vi "VirtualBench_IV Curve (PWS and DMM).vi"() -> ()   [LabVIEW 2015]
doc: "This example demonstrates a voltage sweep and a measurement of the current across the DUT to create an I-V curve."
uses:
  <vilib>/Utility/error.llb/DialogType.ctl
  <vilib>/VirtualBench/_DMM Configure Measurement4.vi
  <vilib>/VirtualBench/_PS Configure Voltage Output0.vi
  <vilib>/VirtualBench/VirtualBench.lvlib
panel:
  in  "Auto Range":i32(ring) items=["Low", "High"]
  in  "PWS Channel":tag="ps/+6V" caption="Channel"
  in  "Current Limit (A)":dbl=0.5 caption="Current Limit (no change)"
  in  "End Voltage (V)":dbl=5.0 caption="Frequency (no change)"
  in  "Start Voltage (V)":dbl caption="Frequency (no change)"
  in  "Number of Steps":i32=10
  in  "VirtualBench Device":tag="VB8012"
  out "Analog Data":cluster{dbl[], dbl[]}(graph)
  # "Power Supply Settings"
  # "DMM Settings"
  # "IV Curve"
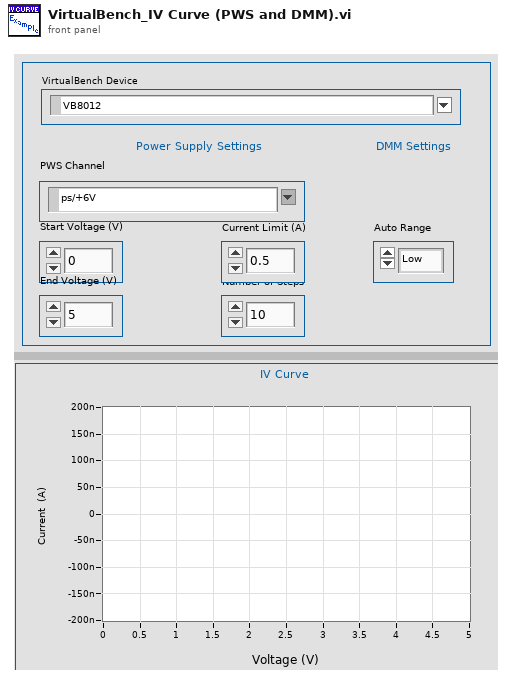
[diagram p1: front panel]
types:
  T1 = typedef "DialogType.ctl" = u16
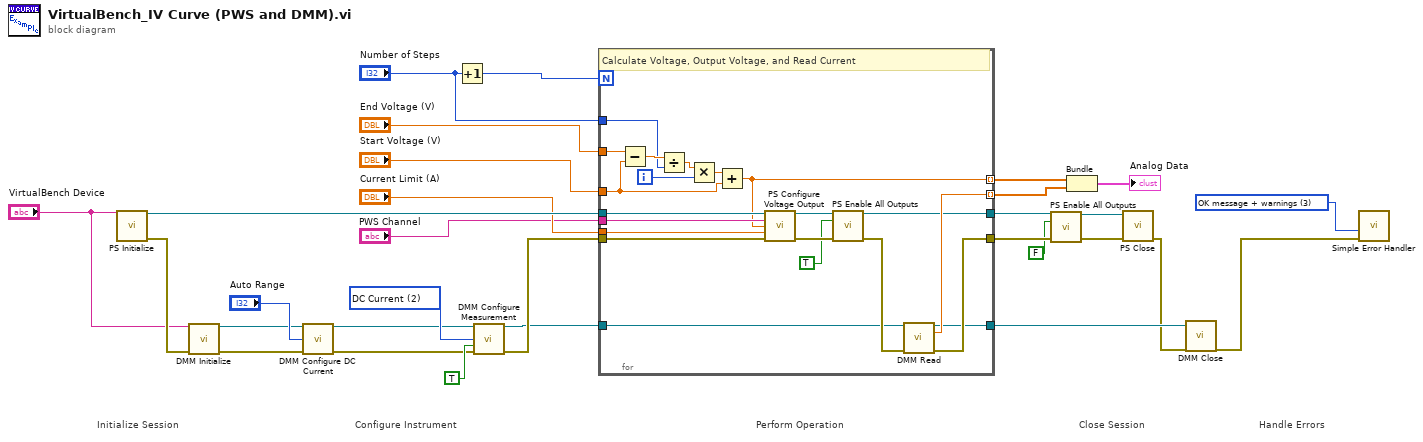
[diagram p0: block diagram]
diagram:
  w12 = 2 items=["DC Volts", "AC Volts", "DC Current", "AC Current", "Resistance", "Diode"] ("Function")
  w29 = T1 3 items=["no dialog", "OK message", "continue or stop message", "OK message + warnings", "continue/stop + warnings"] ("type of dialog (OK msg:1)")
  # "Handle Errors"
  # "Close Session"
  # "Configure Instrument"
  # "Perform Operation"
  # "Initialize Session"
  n1 = call <vilib>:"PS Initialize.vi"("Device Name"="VirtualBench Device") -> ("Instrument Handle Out"=w28:refnum<k21>, "Error Out"=w13:errorcluster)  [unwired: 13 in]
  n2 = call <vilib>:"DMM Initialize.vi"("Device Name"="VirtualBench Device", "Error In"=w13) -> ("Instrument Handle Out"=w1:refnum<k21>, "Error Out"=w2:errorcluster)  [unwired: 12 in]
  n3 = call <vilib>:"DMM Configure DC Current.vi"("Instrument Handle In"=w1, "Auto Range Terminal"="Auto Range", "Error In"=w2) -> ("Instrument Handle Out"=w4:refnum<k21>, "Error Out"=w3:errorcluster)  [unwired: 11 in]
  n4 = Increment(x="Number of Steps") -> (x+1=w30:i32)
  n5 = call-poly <vilib>:"DMM Configure Measurement.vi"("Instrument Handle In"=w4, "Function"=w12, "Auto Range"=TRUE, "Error In"=w3) -> ("Instrument Handle Out"=w7:refnum<k21>, "Error Out"=w14:errorcluster)  [unwired: 10 in]
  n6 = for {
    N: w30 -> [_]
    tunnel: "End Voltage (V)" -> [w48]
    tunnel: "Start Voltage (V)" -> [w47]
    tunnel: w28 -> [w45]
    tunnel: "Current Limit (A)" -> [w44]
    tunnel: "PWS Channel" -> [w40]
    tunnel: [w35] -> w19
    tunnel: [w37] -> w23 mode=indexing
    tunnel: w14 -> [w43]
    tunnel: [w33] -> w18
    tunnel: [w36] -> w22 mode=indexing
    tunnel: "Number of Steps" -> [w38]
    tunnel: [w32] -> w10
    tunnel: w7 -> [w31]
    i -> [w46]
    # "Calculate Voltage, Output Voltage, and Read Current"
    n7 = Subtract(x=w48, y=w47) -> (x-y=w51:dbl)
    n8 = Divide(x=w51, y=w38) -> (x/y=w50:dbl)
    n9 = Multiply(x=w50, y=w46) -> (x*y=w49:dbl)
    n10 = Add(x=w49, y=w47) -> (x+y=w37:dbl)
    n11 = call-poly <vilib>:"PS Configure Voltage Output.vi"("Instrument Handle In"=w45, "Channel"=w40, "Voltage Level"=w37, "Current Limit"=w44, "Error In"=w43) -> ("Instrument Handle Out"=w42:refnum<k21>, "Error Out"=w41:errorcluster)  [unwired: 9 in]
    n12 = call <vilib>:"PS Enable All Outputs.vi"("Instrument Handle In"=w42, "Enable Outputs"=TRUE, "Error In"=w41) -> ("Instrument Handle Out"=w35:refnum<k21>, "Error Out"=w34:errorcluster)  [unwired: 11 in]
    n13 = call <vilib>:"DMM Read.vi"("Instrument Handle In"=w31, "Error In"=w34) -> ("Instrument Handle Out"=w32:refnum<k21>, "Measurement"=w36:dbl, "Error Out"=w33:errorcluster)  [unwired: 11 in]
  }
  n14 = call <vilib>:"PS Enable All Outputs.vi"("Instrument Handle In"=w19, "Enable Outputs"=FALSE, "Error In"=w18) -> ("Instrument Handle Out"=w16:refnum<k21>, "Error Out"=w15:errorcluster)  [unwired: 11 in]
  n15 = Bundle(w23, w22) -> (→"Analog Data":cluster{dbl[], dbl[]})  [unwired: 1 in]
  n16 = call <vilib>:"PS Close.vi"("Instrument Handle In"=w16, "Error In"=w15) -> ("Error Out"=w9:errorcluster)  [unwired: 13 in]
  n17 = call <vilib>:"DMM Close.vi"("Instrument Handle In"=w10, "Error In"=w9) -> ("Error Out"=w8:errorcluster)  [unwired: 13 in]
  n18 = call <vilib>:"Simple Error Handler.vi"("type of dialog (OK msg:1)"=w29, "error in (no error)"=w8) -> ()  [unwired: 3 in, 5 out]
